vi "Get All Topics.vi"(8 "error in (no error)":errorcluster, 11 "TopicLookupTable":refnum<data-value>) -> (0 "error out":errorcluster, 1 "Topic Name":string[](array[string]), 2 "Topic Enqueuers":refnum<class "Message Enqueuer.lvclass">[](array[class]), 3 "TopicLookupTable":refnum<data-value>)   [LabVIEW 2019, in "Mediator.lvlib" / "TopicLookupTable.lvclass"]
doc: "<License>\nCopyright © 2017 Composed Systems, LLC | All rights reserved\nwww.composed.io\n\nAuthor: Ethan Stern <ethan.stern@composed.io>\n\nThis software is provided \"AS IS\" WITHOUT WARRANTIES, either express or implied, AND IS FOR EDUCATIONAL PURPOSES ONLY.\n</License>"
uses:
  <vilib>/gpm_packages/@cs/mva-core/Source/Mediator/TopicLookupTable/TopicLookupTable.lvclass
  <vilib>/ActorFramework/Message Enqueuer/Message Enqueuer.lvclass
  <vilib>/gpm_packages/@cs/mva-core/Source/Mediator/TopicLookupTable/TopicLookupTable.lvclass/TopicLookupTable.ctl
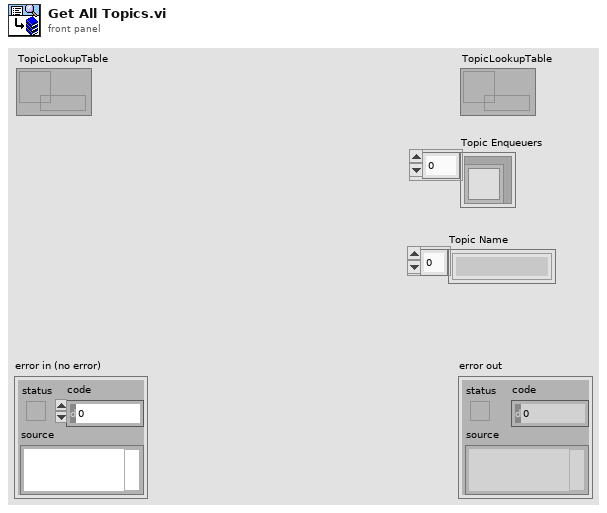
[diagram p1: front panel]
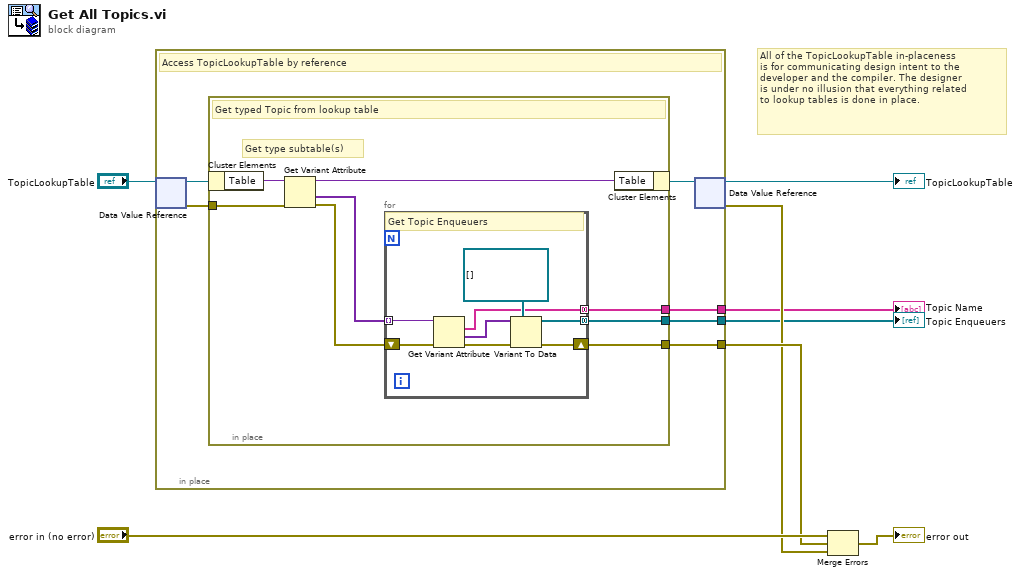
[diagram p0: block diagram]
diagram:
  # "All of the TopicLookupTable in-placeness\nis for communicating design intent to the\ndeveloper and the compiler. The designer\nis under no illusion that everything related\nto lookup tables is done in place."
  n1 = in-place {
    in-place-border: [w14] -> w5
    in-place-border: [w13] -> w2
    in-place-border: [w9] -> w1
    # "Access TopicLookupTable by reference"
    n2 = in-place-dvr #1("TopicLookupTable") -> (w12:refnum<class "TopicLookupTable.lvclass">, w10:errorcluster)
    n3 = in-place {
      in-place-border: [w17] -> w13
      in-place-border: [w16] -> w14
      in-place-border: w10 -> [w22]
      in-place-border: [w15] -> w9
      # "Get type subtable(s)"
      # "Get typed Topic from lookup table"
      n4 = in-place-cluster #2(w12) -> ("Table"=w21:variant)
      n5 = Get Variant Attribute(Variant=w21, error in=w22) -> (duplicate Variant=w19:variant, values=w20:variant[], error out=w18:errorcluster)  [unwired: 2 in, 1 out]
      n6 = for {
        tunnel: w20 -> [w30] mode=indexing
        shift-right: [w26] -> w16
        shift-left: w18 -> [w29]
        tunnel: [w24] -> w17 mode=concatenating
        tunnel: [w23] -> w15 mode=concatenating
        # "Get Topic Enqueuers"
        n7 = Get Variant Attribute(Variant=w30, error in=w29) -> (names=w23:string[], values=w25:variant[], error out=w27:errorcluster)  [unwired: 2 in, 1 out]
        n8 = Variant To Data(error in=w27, type=refnum<class "Message Enqueuer.lvclass">[] [] ("Self Enqueuer"), Variant=w25) -> (data=w24:refnum<class "Message Enqueuer.lvclass">[], error out=w26:errorcluster)
      }
      n9 = in-place-cluster #2("Table"=w19) -> (w11:refnum<class "TopicLookupTable.lvclass">)
    }
    n10 = in-place-dvr #1(w11) -> (→"TopicLookupTable":refnum<data-value>, w4:errorcluster)
  }
  "Topic Enqueuers" <- w2
  "Topic Name" <- w1
  n11 = Merge Errors("error in (no error)", w5, w4) -> (→"error out":errorcluster)
